vi "LoginInteraction.vi"(10 "LoginStatus":T2, 11 "DataIn":T3) -> (2 "NextState":T1, 3 "DataOut":T3)   [LabVIEW 2017]
doc: "SubVI criada para realizar operações de leitura e escrita em arquivo"
uses:
  <vilib>/Utility/file.llb/Write Delimited Spreadsheet (string).vi
  controls/Login - States.ctl
  <vilib>/Utility/file.llb/Read Delimited Spreadsheet (string).vi
  controls/Table.ctl
  controls/GameOption.ctl
  controls/Tabuleiro.ctl
  controls/DataIn.ctl
  controls/LoginStatus.ctl
  MatchDataClasses/MatchData/MatchData.lvclass
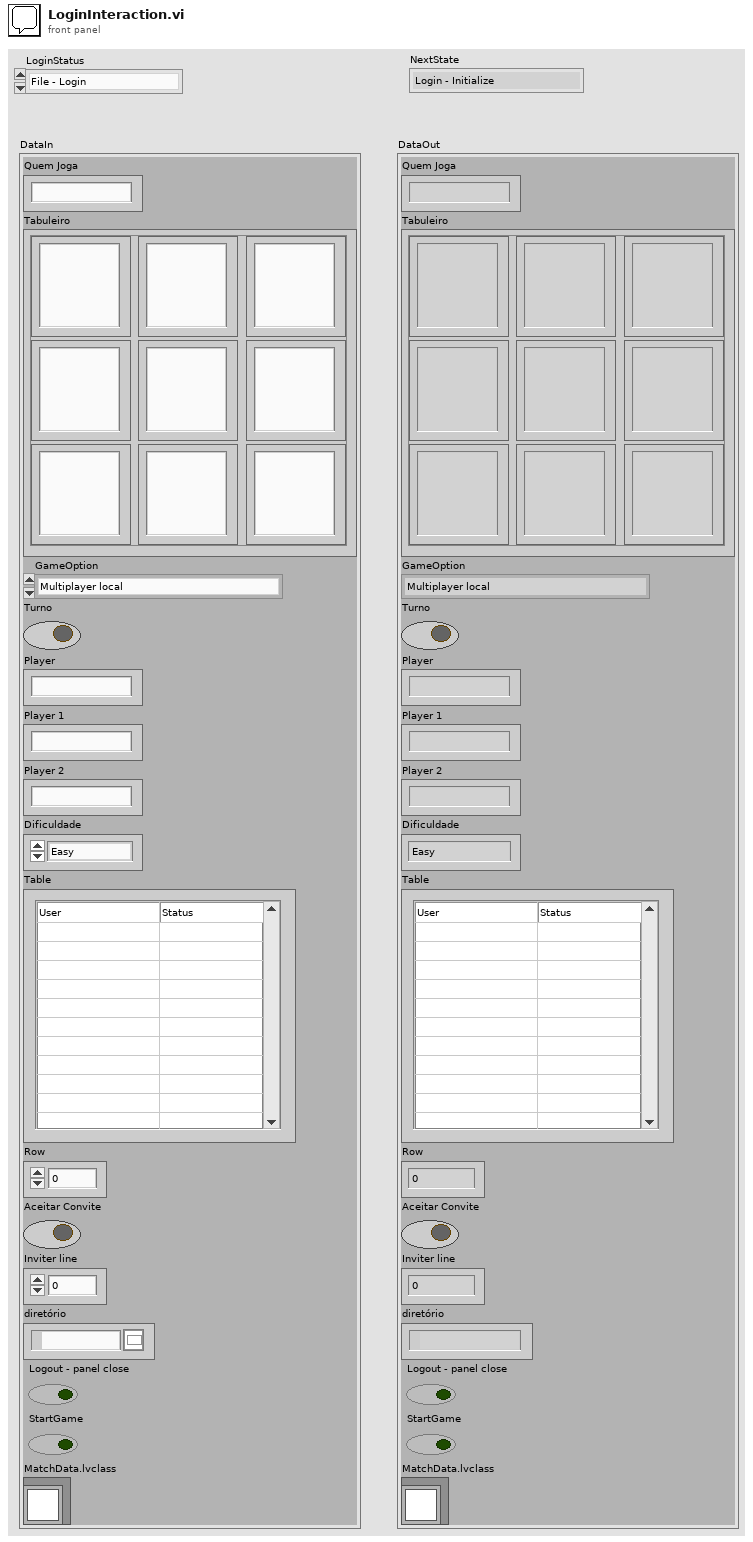
[diagram p1: front panel]
types:
  T1 = typedef "Login - States.ctl" = enum16{"Login - Initialize", "Login - Wait for Event", "Login", "Logout", "Table Refresh", "Invitation"}
  T2 = typedef "LoginStatus.ctl" = enum16{"File - Login", "File - Logout", "File - TableRefresh"}
  T3 = typedef "DataIn.ctl" = cluster{"Quem Joga":string, "Tabuleiro":T4, "GameOption":T5, "Turno":bool, "Player":string, "Player 1":string, "Player 2":string, "Dificuldade":enum16{"Easy", "Medium", "Hard"}, "Table":T6, "Row":u32, "Aceitar Convite":bool, "Inviter line":u32, "diretório":path, "Logout - panel close":bool, "StartGame":bool, "MatchData.lvclass":refnum<class "MatchData.lvclass">}
  T4 = typedef "Tabuleiro.ctl" = cluster{"(0,0)":string, "(1,0)":string, "(0,1)":string, "(1,1)":string, "(2,0)":string, "(1,2)":string, "(2,2)":string, "(0,2)":string, "(2,1) ":string}
  T5 = typedef "GameOption.ctl" = enum16{"Multiplayer local", "Multiplayer remoto", "Single Player", "Wait for Event", "Initialize", "Stop"}
  T6 = typedef "Table.ctl" = string[][]
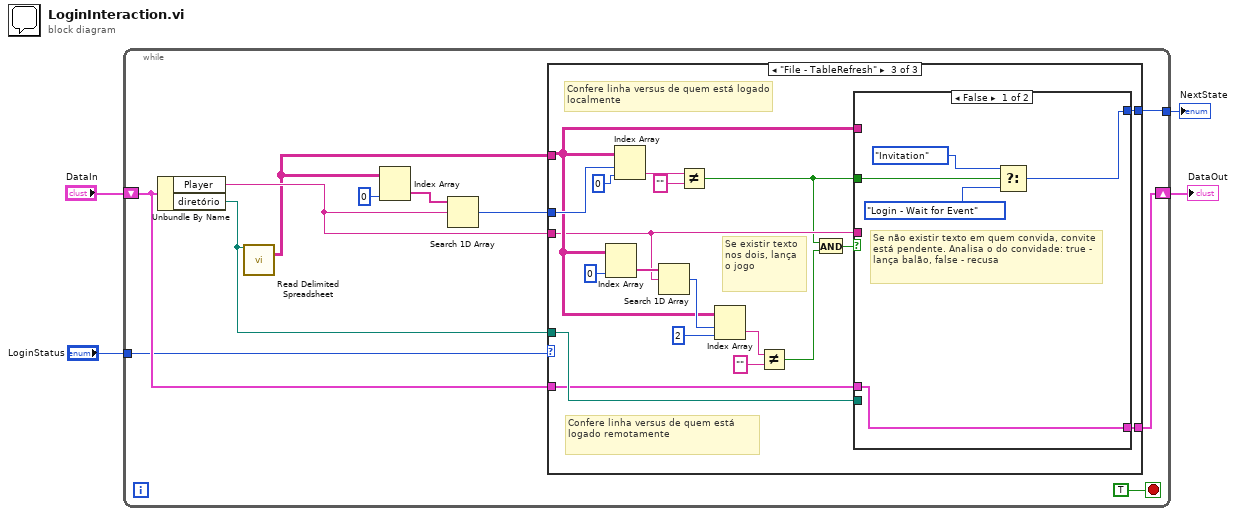
[diagram p0: block diagram]
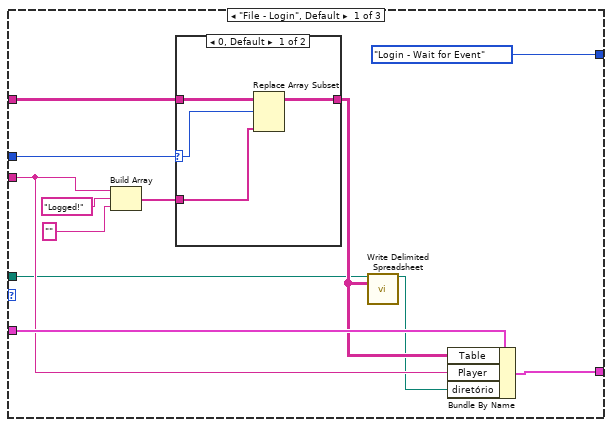
[diagram p2: hidden frame]
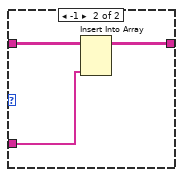
[diagram p3: hidden frame]
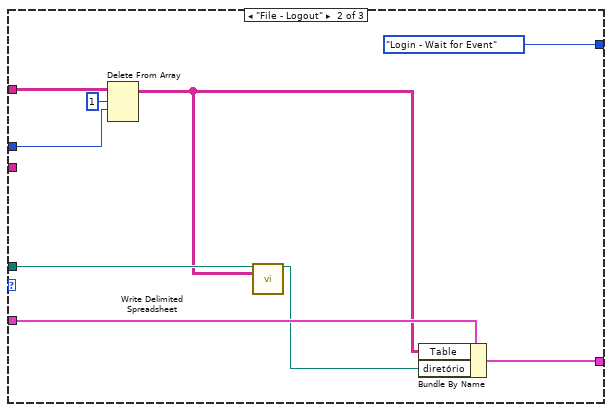
[diagram p4: hidden frame]
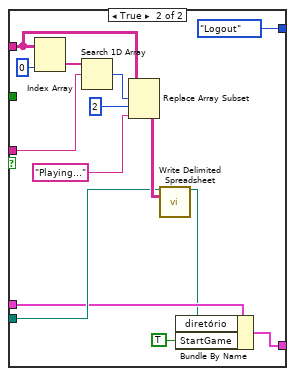
[diagram p5: hidden frame]
diagram:
  n1 = while {
    tunnel: "LoginStatus" -> [w7]
    shift-right: [w8] -> w3
    shift-left: "DataIn" -> [w9]
    tunnel: [w6] -> w1
    stop <- TRUE stop-if-true
    n2 = Unbundle By Name(w9) -> ("Player"=w12:string, "diretório"=w10:path)
    n3 = call-poly <vilib>:"Read Delimited Spreadsheet.vi"("file path (dialog if empty)"=w10) -> ("all rows"=w11:string[][])  [unwired: 9 in, 5 out]
    n4 = Index Array(array=w11, index (col)=0 ("disabled index (col)")) -> (element=w14:string[])  [unwired: 1 in]
    n5 = Search 1D Array(1D array=w14, element=w12) -> (index of element=w13:i32)  [unwired: 1 in]
    n6 = case shown="\"File - TableRefresh\"" w7 {
      tunnel: w13 -> [w25 w42 w62]
      tunnel: w12 -> [w20 _ w49]
      tunnel: w11 -> [w24 w43 w50]
      tunnel: w10 -> [w19 w40 w48]
      tunnel: w9 -> [w22 w39 w47]
      tunnel: [w18 w36 w46] -> w8
      tunnel: [Login_-_States."Login - Wait for Event" Login_-_States."Login - Wait for Event" w45] -> w6
      frame "File - Login", Default {
        n7 = Build Array(w20, "Logged!" ("string"), "" ("string")) -> (w23:string[])
        n8 = case shown="0, Default" w25 {
          selector: w25 -> [w30 _]
          tunnel: w23 -> [w28 w32]
          tunnel: w24 -> [w31 w34]
          tunnel: [w29 w33] -> w21
          frame 0, Default {
            n9 = Replace Array Subset(array=w31, new element=w28, index (row)=w30) -> (w29:string[][])  [unwired: 1 in]
          }
          frame -1 {
            n10 = Insert Into Array(array=w34, new element=w32) -> (w33:string[][])  [unwired: 2 in]
          }
        }
        n11 = call-poly <vilib>:"Write Delimited Spreadsheet.vi"("file path (dialog if empty)"=w19, "2D data"=w21) -> ("new file path (Not A Path if cancelled)"=w16:path)  [unwired: 12 in, 1 out]
        n12 = Bundle By Name(cluster=w22, "Table"=w21, "Player"=w20, "diretório"=w16) -> (w18:T3)
      }
      frame "File - Logout" {
        n13 = Delete From Array(array=w43, length=1, index (row)=w42) -> (array with subset deleted=w37:string[][])  [unwired: 1 in, 1 out]
        n14 = call-poly <vilib>:"Write Delimited Spreadsheet.vi"("file path (dialog if empty)"=w40, "2D data"=w37) -> ("new file path (Not A Path if cancelled)"=w38:path)  [unwired: 12 in, 1 out]
        n15 = Bundle By Name(cluster=w39, "Table"=w37, "diretório"=w38) -> (w36:T3)
      }
      frame "File - TableRefresh" {
        # "Confere linha versus de quem está logado localmente"
        # "Confere linha versus de quem está logado remotamente"
        # "Se existir texto nos dois, lança o jogo"
        n16 = Index Array(array=w50, index (col)=0 ("disabled index (col)")) -> (element=w59:string[])  [unwired: 1 in]
        n17 = Index Array(array=w50, index (row)=w62, index (col)=0 ("disabled index (col)")) -> (element=w56:string)
        n18 = Search 1D Array(1D array=w59, element=w49) -> (index of element=w58:i32)  [unwired: 1 in]
        n19 = Not Equal?(x=w56, y="") -> (x != y?=w44:bool)
        n20 = Index Array(array=w50, index (row)=w58, index (col)=2 ("disabled index (col)")) -> (element=w53:string)
        n21 = Not Equal?(x=w53, y="") -> (x != y?=w52:bool)
        n22 = And(x=w44, y=w52) -> (x .and. y?=w51:bool)
        n23 = case shown="False" w51 {
          tunnel: w50 -> [_ w68]
          tunnel: w49 -> [_ w76]
          tunnel: w48 -> [_ w74]
          tunnel: w47 -> [w63 w73]
          tunnel: [w63 w71] -> w46
          tunnel: [w64 Login_-_States."Logout"] -> w45
          tunnel: w44 -> [w67 _]
          frame False {
            # "Se não existir texto em quem convida, convite está pendente. Analisa o do convidade: true - lança balão, false - recusa"
            n24 = Select(t=Login_-_States."Invitation", s=w67, f=Login_-_States."Login - Wait for Event") -> (s? t:f=w64:T1)
          }
          frame True {
            n25 = Index Array(array=w68, index (col)=0 ("index (row)")) -> (element=w77:string[])  [unwired: 1 in]
            n26 = Search 1D Array(1D array=w77, element=w76) -> (index of element=w80:i32)  [unwired: 1 in]
            n27 = Replace Array Subset(array=w68, new element="Playing..." ("new element/subarray"), index (row)=w80, index (col)=2 ("disabled index (col)")) -> (w75:string[][])
            n28 = call-poly <vilib>:"Write Delimited Spreadsheet.vi"("file path (dialog if empty)"=w74, "2D data"=w75) -> ("new file path (Not A Path if cancelled)"=w72:path)  [unwired: 12 in, 1 out]
            n29 = Bundle By Name(cluster=w73, "diretório"=w72, "StartGame"=TRUE) -> (w71:T3)
          }
        }
      }
    }
  }
  "DataOut" <- w3
  "NextState" <- w1
